vi "UDT_ErrorMonitor_HandleError.vi"() -> (3 "Unit Test Framework Results":T1)   [LabVIEW 2017]
doc: "Use this template to create a user-defined test VI. Define your test requirements and wire the results to the <b>Result (Test)</b> control. Do not modify the <b>Unit Test Framework Results</b> indicator."
uses:
  <vilib>/utf/common/utf_test_result_troll.ctl
  <vilib>/utf/common/utf_test_result.ctl
  <vilib>/utf/common/utf_test_result_failure.ctl
  <vilib>/utf/common/utf_test_comparison_operators.ctl
  <vilib>/utf/common/utf_vi_tag.ctl
  RT/ErrorMonitor/Queue/TypeDefs/queueFGVState.ctl
  RT/ErrorMonitor/ErrorMonitor.lvlib
  <vilib>/Control Software Solutions Ltd/UTF Helper/Unit Test Helper.lvlib
  <vilib>/utf/NI_UnitTestFramework.lvlib
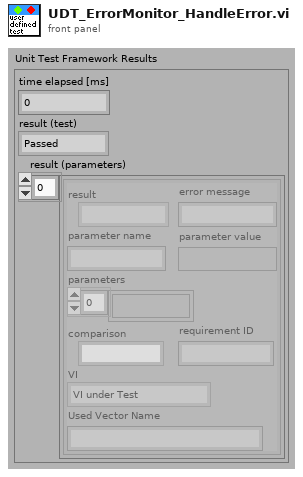
[diagram p1: front panel]
types:
  T1 = typedef "NI_UnitTestFramework.lvlib/utf_test_result_troll.ctl" = cluster{"time elapsed [ms]":u32, "result (test)":T2, "result (parameters)":T3[]}
  T2 = typedef "NI_UnitTestFramework.lvlib/utf_test_result.ctl" = enum16{"Passed", "Failed", "Error", "Skipped", "Not Processed"}
  T3 = typedef "NI_UnitTestFramework.lvlib/utf_test_result_failure.ctl" = cluster{"result":T2, "error message":string, "parameter name":string, "parameter value":variant, "parameters":variant[], "comparison":T4, "requirement ID":string, "VI":T5, "Used Vector Name":string}
  T4 = typedef "NI_UnitTestFramework.lvlib/utf_test_comparison_operators.ctl" = enum16{"=", "!=", ">", ">=", "<", "<=", "range", "symmetric tolerance", "asymmetric tolerance", "string contains", "string not contain", "array size", "string length", "array range", "by element", "array range (limit array)", "user-defined", "array contains", "array not contain", "vector length", "= (elm)", "!= (elm)", "= (case insensitive)", "!= (case insensitive)"}
  T5 = typedef "NI_UnitTestFramework.lvlib/utf_vi_tag.ctl" = enum16{"Setup VI", "VI under Test", "Teardown VI"}
  T6 = typedef "ErrorMonitor.lvlib/queueFGVState.ctl" = enum16{"obtain", "enqueue low priority", "enqueue high priority", "dequeue", "release"}
  T7 = typedef "ErrorMonitor.lvlib/message.ctl" = cluster{"calling module":string, "message":string, "Data":variant}
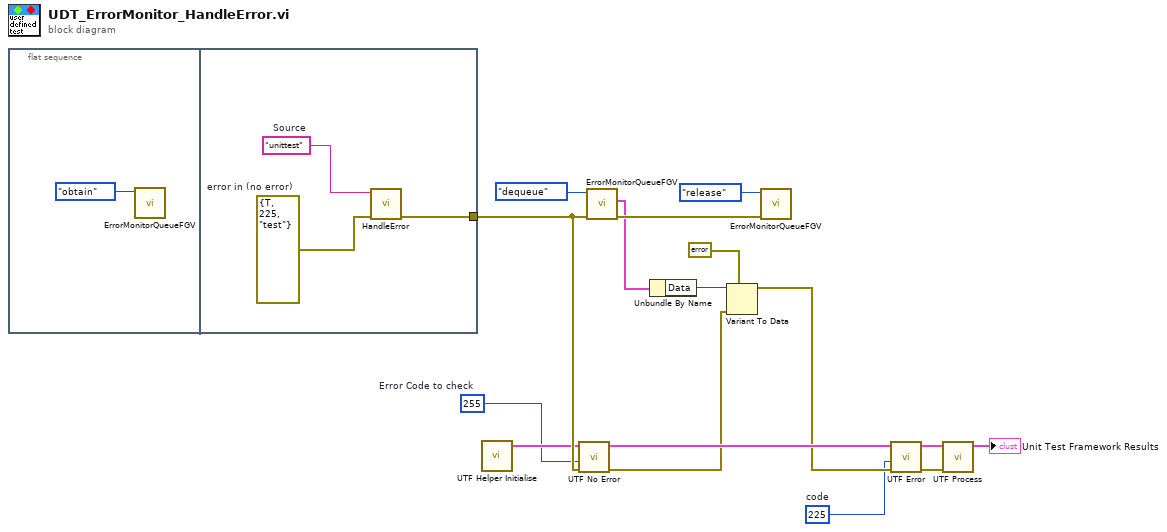
[diagram p0: block diagram]
diagram:
  w1 = 225  # code
  w2 = 255  # Error Code to check
  n1 = flat-sequence {
    tunnel: [w18] -> w12
    frame #0 {
      n2 = call "ErrorMonitorQueueFGV.vi"("Enum"=queueFGVState."obtain") -> ()  [unwired: 9 in, 2 out]
    }
    frame #1 {
      w19 = errorcluster {"status"=TRUE, "code"=225, "source"="test"}  # error in (no error)
      w20 = "unittest"  # Source
      n3 = call "HandleError.vi"("error in (no error)"=w19, "Source"=w20) -> ("error out"=w18:errorcluster)  [unwired: 9 in]
    }
  }
  n4 = call <vilib>:"UTF Helper Initialise.vi"() -> ("results array"=w11:T3[])  [unwired: 10 in, 1 out]
  n5 = call <vilib>:"UTF No Error.vi"("error in (no error)"=w12, "Error Code to check"=w2, "Input Results"=w11) -> ("error out"=w6:errorcluster, "Output Results"=w7:T3[])  [unwired: 7 in]
  n6 = call "ErrorMonitorQueueFGV.vi"("error in (no error)"=w12, "Enum"=queueFGVState."dequeue") -> ("error out"=w14:errorcluster, "message out"=w10:T7)  [unwired: 8 in]
  n7 = Unbundle By Name(w10) -> ("Data"=w9:variant)
  n8 = Variant To Data(error in=w6, type=errorcluster {"status"=FALSE, "code"=0, "source"=""} ("error constant"), Variant=w9) -> (data=w5:errorcluster)  [unwired: 1 out]
  n9 = call "ErrorMonitorQueueFGV.vi"("error in (no error)"=w14, "Enum"=queueFGVState."release") -> ()  [unwired: 8 in, 2 out]
  n10 = call <vilib>:"UTF Error.vi"("error in (no error)"=w5, "Expected Error Code"=w1, "Input Results"=w7) -> ("error out"=w3:errorcluster, "Output Results"=w4:T3[])  [unwired: 7 in]
  n11 = call <vilib>:"UTF Process.vi"("error in (no error)"=w3, "results array"=w4) -> ("Unit Test Framework Results"=→"Unit Test Framework Results":T1)  [unwired: 9 in]
